vi "Periodic Tasks.vi"(8 "error in":errorcluster) -> ()   [LabVIEW 2018]
doc: "This VI runs in parallel to other tasks. It can contain as many user-defined periodic loops as you need. These can carry out PID or other sorts of timed response."
uses:
  <vilib>/Rock Robotics/WPI/Solenoid/WPI_SolenoidValue.ctl
  Swerve/SwerveGlobals.vi
  <vilib>/Rock Robotics/Network Tables/NT Write String.vi
  <vilib>/Rock Robotics/WPI/Solenoid/WPI_SolenoidSetEnum.vi
  navx-mxp/labview/navX Library v2/navX Library v2.lvlib
panel:
  out "navX axes":T1
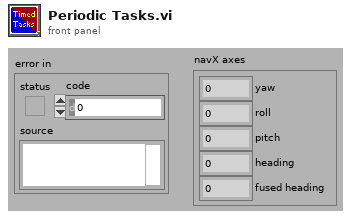
[diagram p1: front panel]
types:
  T1 = cluster{"yaw":dbl, "roll":dbl, "pitch":dbl, "heading":dbl, "fused heading":dbl}
  T2 = typedef "WPI_SwitchDevRef.ctl" = cluster{"DevStatus":errorcluster, "DIO Channel":T3, "CntIndex":T4, "Normally Closed":bool}
  T3 = typedef "FPGA_DIOChannel.ctl" = enum8{"DIO 0", "DIO 1", "DIO 2", "DIO 3", "DIO 4", "DIO 5", "DIO 6", "DIO 7", "DIO 8", "DIO 9", "DIO MXP 0", "DIO MXP 1", "DIO MXP 2", "DIO MXP 3", "DIO MXP 4", "DIO MXP 5", "DIO MXP 6", "DIO MXP 7", "DIO MXP 8", "DIO MXP 9", "DIO MXP 10", "DIO MXP 11", "DIO MXP 12", "DIO MXP 13", "DIO MXP 14", "DIO MXP 15", "SPI Port CS1", "SPI Port CS2", "SPI Port CS3", "SPI Port MISO", "SPI Port MOSI", "Invalid"}
  T4 = typedef "FPGA_CounterCtrSystemIndex.ctl" = enum8{"Ctr 0", "Ctr 1", "Ctr 2", "Ctr 3", "Ctr 4", "Ctr 5", "Ctr 6", "Ctr 7", "Invalid"}
  T5 = typedef "navX Library v2.lvlib/Z900_navX_DeviceTypeDef.ctl" = cluster{"Interface":cluster{"Protocol":T6, "Update Rate (4Hz-100Hz)":u8, "navX Open TypeDef":variant}, "Notify Packet":refnum<notifier>, "Loop VI Refnum":refnum<vi>, "Ready to Close Occurrence Refnum":refnum<k4>}
  T6 = typedef "navX Library v2.lvlib/Z900_navX_ProtocolTypeDef.ctl" = enum16{"SERIAL", "I2C", "SPI"}
  T7 = typedef "WPI_AnalogChannelDevRef.ctl" = cluster{"DevStatus":errorcluster, "Analog Channel":T8}
  T8 = typedef "FPGA_AIChannel.ctl" = enum8{"AI 0", "AI 1", "AI 2", "AI 3", "AI MXP 0", "AI MXP 1", "AI MXP 2", "AI MXP 3", "Invalid"}
  T9 = typedef "WPI_MotorControlDeviceRef.ctl" = cluster{"DeviceStatus":errorcluster, "Type":T10, "PWM":cluster{"PWM Channel":T11, "DeadBand":T12}, "CAN":cluster{"Device Number":u8, "SetOutput VI Ref":variant, "GetOutput VI Ref":variant, "Enable VI Ref":variant, "Disable VI Ref":variant, "Data":variant}, "Invert":bool, "DIO PWM":cluster{"PWM \"Enable\" Channel":T11, "DIOChannel":T3, "PWM Rate":dbl}}
  T10 = typedef "WPI_MotorControlType.ctl" = enum16{"PWM", "CAN", "DIO PWM"}
  T11 = typedef "FPGA_DIOPWMChannel.ctl" = enum8{"PWM 0", "PWM 1", "PWM 2", "PWM 3", "PWM 4", "PWM 5", "PWM 6", "PWM 7", "PWM 8", "PWM 9", "PWM MXP 0", "PWM MXP 1", "PWM MXP 2", "PWM MXP 3", "PWM MXP 4", "PWM MXP 5", "PWM MXP 6", "PWM MXP 7", "PWM MXP 8", "PWM MXP 9", "Invalid"}
  T12 = typedef "WPI_PWMDeadband.ctl" = cluster{"Name":string, "maxPositivePwm":i32, "minPositivePwm":i32, "centerPwm":i32, "maxNegativePwm":i32, "minNegativePwm":i32, "angularRange":u16}
  T13 = typedef "WPI_EncoderDevRef.ctl" = cluster{"DevStatus":errorcluster, "EncoderIndex":T14, "CounterIndex":T4, "DistancePerCount":dbl, "Decoding Type":T15}
  T14 = typedef "FPGA_EncoderIdx.ctl" = enum8{"Enc 0", "Enc 1", "Enc 2", "Enc 3", "Enc 4", "Enc 5", "Enc 6", "Enc 7", "Invalid"}
  T15 = typedef "WPI_EncoderType.ctl" = enum16{"1x", "2x", "4x"}
  T16 = typedef "WPI_SolenoidDevRef.ctl" = cluster{"DevStatus":errorcluster, "Pneumatics Control Module":u8, "Forward Solenoid Channel":T17, "Reverse Solenoid Channel":T17}
  T17 = typedef "WPI_SolenoidChannel.ctl" = enum8{"Solenoid 0", "Solenoid 1", "Solenoid 2", "Solenoid 3", "Solenoid 4", "Solenoid 5", "Solenoid 6", "Solenoid 7", "Invalid"}
  T18 = typedef "WPI_SolenoidValue.ctl" = enum16{"Off", "On", "Forward", "Reverse"}
  T19 = cluster{"Yaw":dbl, "Roll":dbl, "Pitch":dbl, "Heading":dbl, "Fused Heading":dbl}
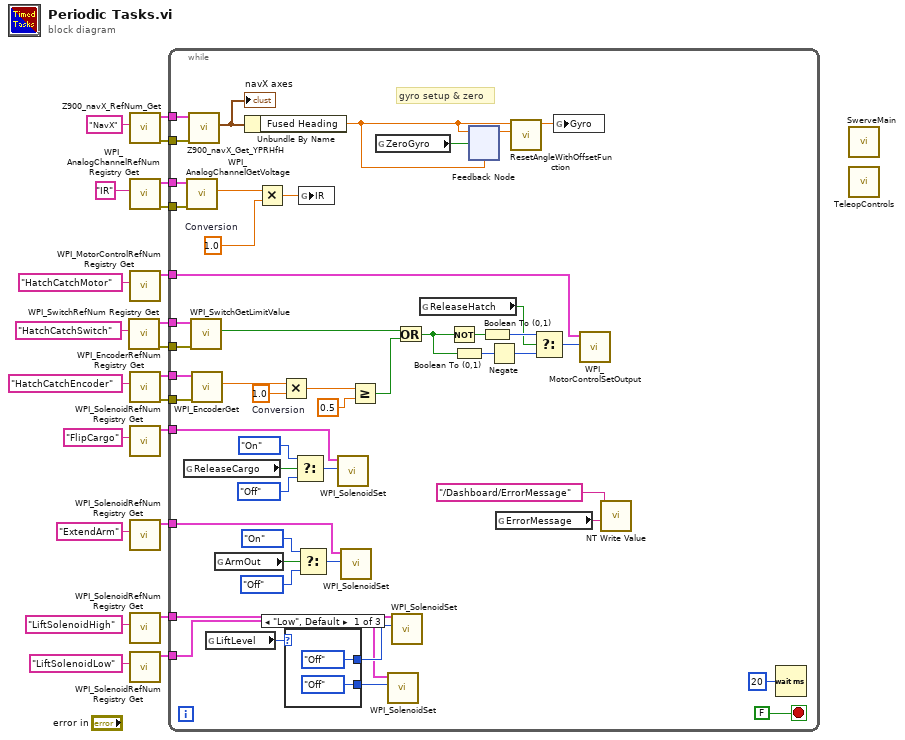
[diagram p0: block diagram]
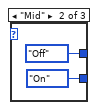
[diagram p2: hidden frame]
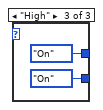
[diagram p3: hidden frame]
diagram:
  n1 = call <vilib>:"WPI_SwitchRefNum Registry Get.vi"("refnum name"="HatchCatchSwitch") -> ("error out"=w1:errorcluster, "SwitchDevRef"=w2:T2)  [unwired: 9 in]
  n2 = call "Z900_navX_RefNum_Get.vi"("refnum name"="NavX") -> ("error out"=w3:errorcluster, "navX Device"=w21:T5)  [unwired: 9 in]
  n3 = call <vilib>:"WPI_AnalogChannelRefNum Registry Get.vi"("refnum name"="IR") -> ("error out"=w18:errorcluster, "AIDeviceRef"=w19:T7)  [unwired: 9 in]
  n4 = call <vilib>:"WPI_MotorControlRefNum Registry Get.vi"("refnum name"="HatchCatchMotor") -> ("MotorControlDevRef"=w17:T9)  [unwired: 9 in, 1 out]
  n5 = call <vilib>:"WPI_EncoderRefNum Registry Get.vi"("refnum name"="HatchCatchEncoder") -> ("error out"=w9:errorcluster, "EncoderDevRef"=w10:T13)  [unwired: 9 in]
  n6 = call <vilib>:"WPI_SolenoidRefNum Registry Get.vi"("refnum name"="FlipCargo") -> ("SolenoidDevRef"=w6:T16)  [unwired: 9 in, 1 out]
  n7 = call <vilib>:"WPI_SolenoidRefNum Registry Get.vi"("refnum name"="ExtendArm") -> ("SolenoidDevRef"=w5:T16)  [unwired: 9 in, 1 out]
  n8 = call <vilib>:"WPI_SolenoidRefNum Registry Get.vi"("refnum name"="LiftSolenoidHigh") -> ("SolenoidDevRef"=w16:T16)  [unwired: 9 in, 1 out]
  n9 = call <vilib>:"WPI_SolenoidRefNum Registry Get.vi"("refnum name"="LiftSolenoidLow") -> ("SolenoidDevRef"=w15:T16)  [unwired: 9 in, 1 out]
  n10 = while {
    tunnel: w21 -> [w65]
    tunnel: w19 -> [w64]
    tunnel: w18 -> [w62]
    tunnel: w17 -> [w30]
    tunnel: w16 -> [w56]
    tunnel: w15 -> [w57]
    tunnel: w10 -> [w55]
    tunnel: w9 -> [w54]
    tunnel: w6 -> [w41]
    tunnel: w5 -> [w36]
    tunnel: w3 -> [w34]
    tunnel: w2 -> [w33]
    tunnel: w1 -> [w32]
    stop <- FALSE stop-if-true
    w52 = 1.0  # Conversion
    w61 = 1.0  # Conversion
    # "gyro setup & zero"
    n11 = global read "SwerveGlobals.vi" "ReleaseCargo"() -> (w45:bool)
    n12 = call <vilib>:"WPI_AnalogChannelGetVoltage.vi"("error in (no error)"=w62, "AIDeviceRef"=w64) -> ("Voltage"=w63:dbl)  [unwired: 7 in, 2 out]
    n13 = call "Z900_navX_Get_YPRHfH.vi"("error in (no error)"=w34, "navX Device"=w65) -> ("YRPHfH"=w68:T19)  [unwired: 6 in, 3 out]
    "navX axes" <- w68
    n14 = call <vilib>:"WPI_SwitchGetLimitValue.vi"("error in (no error)"=w32, "SwitchDevRef"=w33) -> ("Switch Pressed"=w31:bool)  [unwired: 7 in, 2 out]
    n15 = call <vilib>:"WPI_EncoderGet.vi"("error in (no error)"=w54, "EncoderDevRef"=w55) -> ("Distance"=w53:dbl)  [unwired: 4 in, 5 out]
    n16 = global read "SwerveGlobals.vi" "LiftLevel"() -> (w60:enum16{"Low", "Mid", "High"})
    n17 = global read "SwerveGlobals.vi" "ArmOut"() -> (w40:bool)
    n18 = Unbundle By Name(w68) -> ("Fused Heading"=w35:dbl)
    n19 = Multiply(x=w63, y=w61) -> (x*y=w48:dbl)
    n20 = Multiply(x=w53, y=w52) -> (x*y=w51:dbl)
    n21 = case shown="\"Low\", Default" w60 {
      tunnel: [WPI_SolenoidValue."Off" ("Value") WPI_SolenoidValue."Off" ("Value") WPI_SolenoidValue."On" ("Value")] -> w59
      tunnel: [WPI_SolenoidValue."Off" ("Value") WPI_SolenoidValue."On" ("Value") WPI_SolenoidValue."On" ("Value")] -> w58
      frame "Low", Default {
      }
      frame "Mid" {
      }
      frame "High" {
      }
    }
    n22 = Select(t=WPI_SolenoidValue."On" ("Value"), s=w45, f=WPI_SolenoidValue."Off") -> (s? t:f=w42:T18)
    n23 = Select(t=WPI_SolenoidValue."On" ("Value"), s=w40, f=WPI_SolenoidValue."Off") -> (s? t:f=w37:T18)
    n24 = global write "SwerveGlobals.vi" "IR"(w48) -> ()
    n25 = call-poly <vilib>:"WPI_SolenoidSet.vi"("Value"=w42, "SolenoidDevRef"=w41) -> ()  [unwired: 8 in, 2 out]
    n26 = call-poly <vilib>:"WPI_SolenoidSet.vi"("Value"=w37, "SolenoidDevRef"=w36) -> ()  [unwired: 8 in, 2 out]
    n27 = Greater Or Equal?(x=w51, y=0.5) -> (x >= y?=w49:bool)
    n28 = global read "SwerveGlobals.vi" "ZeroGyro"() -> (w66:bool)
    n29 = call-poly <vilib>:"WPI_SolenoidSet.vi"("Value"=w58, "SolenoidDevRef"=w57) -> ()  [unwired: 8 in, 2 out]
    n30 = call-poly <vilib>:"WPI_SolenoidSet.vi"("Value"=w59, "SolenoidDevRef"=w56) -> ()  [unwired: 8 in, 2 out]
    n31 = Or(x=w31, y=w49) -> (x .or. y?=w27:bool)
    n32 = global read "SwerveGlobals.vi" "ReleaseHatch"() -> (w24:bool)
    n33 = Not(x=w27) -> (.not. x?=w29:bool)
    n34 = Boolean To (0,1)(Boolean=w27) -> (0, 1=w28:i16)
    n35 = feedback-in #1(w35, w66) -> ()
    n36 = feedback #1(w35) -> (w69:dbl)
    n37 = Boolean To (0,1)(Boolean=w29) -> (0, 1=w25:i16)
    n38 = Negate(x=w28) -> (-x=w26:i16)
    n39 = global read "SwerveGlobals.vi" "ErrorMessage"() -> (w47:string)
    n40 = call "ResetAngleWithOffsetFunction.vi"("Offset"=w69, "AngleInput"=w35) -> ("AngleOutput"=w67:dbl)  [unwired: 9 in]
    n41 = Select(t=w25, s=w24, f=w26) -> (s? t:f=w23:i16)
    n42 = global write "SwerveGlobals.vi" "Gyro"(w67) -> ()
    n43 = call <vilib>:"WPI_MotorControlSetOutput.vi"("Output"=w23, "MotorControlDevRef"=w30) -> ()  [unwired: 7 in, 3 out]
    n44 = call-poly <vilib>:"NT Write Value.vi"("String"=w47, "Name"="/Dashboard/ErrorMessage") -> ()  [unwired: 9 in, 1 out]
    n45 = Wait (ms)(milliseconds to wait=u32 20) -> ()  [unwired: 1 out]
  }
  n46 = call "SwerveMain.vi"() -> ()  [unwired: 12 in]
  n47 = call "TeleopControls.vi"() -> ()  [unwired: 16 in]
